vi "test-linear-filter-test-03-funcB.vi"(11 "Input":dbl) -> (3 "Output":dbl)   [LabVIEW 2019]
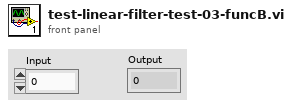
[diagram p1: front panel]
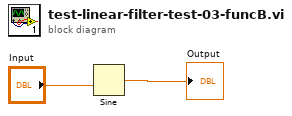
[diagram p0: block diagram]
diagram:
  n1 = Sine(x="Input") -> (sin(x)=→"Output":dbl)
